vi "Persist New Entity.vi"(8 "error in (no error)":errorcluster, 10 "New Entity":refnum<class "Entity.lvclass">, 11 "Entity Manager in":refnum<class "Entity Manager.lvclass">) -> (0 "error out":errorcluster, 2 "Entity":refnum<class "Entity.lvclass">, 3 "Entity Manager out":refnum<class "Entity Manager.lvclass">)   [LabVIEW 2020, in "Conditu2.lvlib" / "Entity Manager.lvclass"]
uses:
  Entity Manager.lvclass
  Entity/Entity.lvclass
  Entity/Entity.lvclass/Entity.ctl
  Columns/ID/ID.lvclass/ID.ctl
  Entity/Update ID.vi
  Columns/ID/Set.vi
  Unit Of Work Session/Unit Of Work Session.lvclass
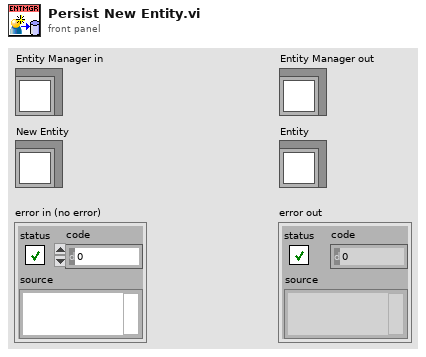
[diagram p1: front panel]
types:
  T1 = typedef "Conditu2.lvlib/Entity ID.ctl" = i64
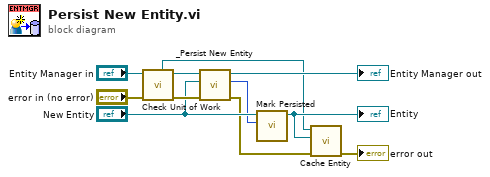
[diagram p0: block diagram]
diagram:
  n1 = call "Check Unit of Work.vi"("error in (no error)"="error in (no error)", "Entity Manager in"="Entity Manager in") -> ("error out"=w11:errorcluster, "Entity Manager out"=w5:refnum<class "Entity Manager.lvclass">, "Unit Of Work"=w1:refnum<class "Unit Of Work Session.lvclass">)  [unwired: 7 in]
  n2 = call "_Persist New Entity.vi"("error in (no error)"=w11, "New Entity"="New Entity", "Entity Manager in"=w5) -> ("error out"=w3:errorcluster, "Entity ID"=w8:T1, "Entity Manager out"=→"Entity Manager out":refnum<class "Entity Manager.lvclass">)  [unwired: 6 in]
  n3 = call "Mark Persisted.vi"("Entity ID"=w8, "Entity in"="New Entity") -> ("Entity out"=w4:refnum<class "Entity.lvclass">)  [unwired: 9 in]
  "Entity" <- w4
  n4 = call "Cache Entity.vi"("error in (no error)"=w3, "Conditum:Entity"=w4, "Unit Of Work in"=w1) -> ("error out"=→"error out":errorcluster)  [unwired: 8 in]
